vi "Create.vi"(6 "commandTimeout":i32, 8 "error in (no error)":errorcluster, 9 "DynamicParameters":refnum<class "DynamicParameters.lvclass">, 10 "tableName":string, 11 "SqlMapper in":refnum<class "SqlMapper.lvclass">) -> (0 "error out":errorcluster, 2 "id":variant, 3 "SqlMapper out":refnum<class "SqlMapper.lvclass">)   [LabVIEW 2020, in "ORM.lvlib" / "SqlMapper.lvclass"]
uses:
  SqlMapper.lvclass
  SqlMapper.lvclass/SqlMapper.ctl
  DbConnection/DbConnection.lvclass
  DynamicParameters/DynamicParameters.lvclass
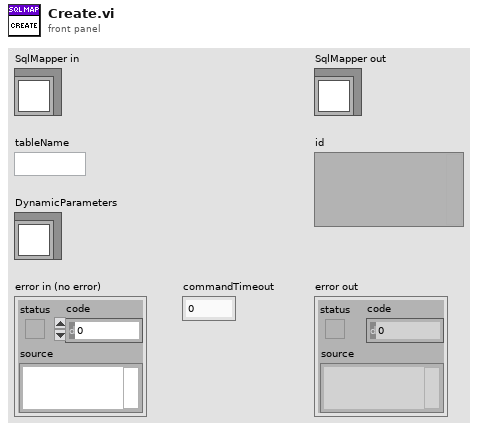
[diagram p1: front panel]
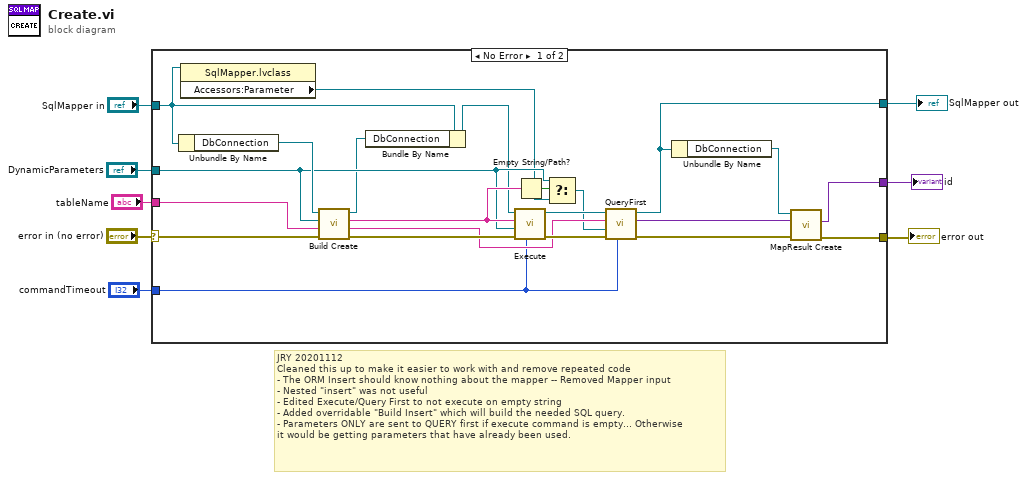
[diagram p0: block diagram]
diagram:
  # "JRY 20201112\nCleaned this up to make it easier to work with and remove repeated code\n- The ORM Insert should know nothing about the mapper -- Removed Mapper input\n- Nested \"insert\" was not useful\n- Edited Execute/Query First to not execute on empty string\n- Added overridable \"Build Insert\" which will build the needed SQL query.\n- Parameters ONLY are sent to QUERY first if execute command is empty... Otherwise\nit would be getting parameters that have already been used."
  n1 = case shown="No Error" "error in (no error)" {
    selector: "error in (no error)" -> [w30 w31]
    tunnel: "SqlMapper in" -> [w10 w32]
    tunnel: [w12 w32] -> w6
    tunnel: "DynamicParameters" -> [w16 _]
    tunnel: [w23 _] -> w4
    tunnel: [w21 w31] -> w3
    tunnel: "commandTimeout" -> [w15 _]
    tunnel: "tableName" -> [w20 _]
    frame No Error {
      n2 = Unbundle By Name(w10) -> ("DbConnection"=w25:refnum<class "DbConnection.lvclass">)
      n3 = property class="SqlMapper.lvclass"(reference=w10) -> ("Accessors:Parameter"=w9:refnum<class "DynamicParameters.lvclass">)  [unwired: 1 in, 2 out]
      n4 = call-dynamic "Build Create.vi"("error in (no error)"=w30, "tableName"=w20, "DynamicParameters in"=w16, "DbConnection in"=w25) -> ("error out"=w29:errorcluster, "LastIdentityQuery"=w26:string, "InsertStatement"=w19:string, "DbConnection out"=w13:refnum<class "DbConnection.lvclass">)  [unwired: 4 in]
      n5 = Bundle By Name(cluster=w10, "DbConnection"=w13) -> (w14:refnum<class "SqlMapper.lvclass">)
      n6 = call-dynamic "Execute.vi"("commandTimeout"=w15, "error in (no error)"=w29, "DynamicParameters"=w16, "sql"=w19, "SqlMapper in"=w14) -> ("error out"=w28:errorcluster, "SqlMapper out"=w27:refnum<class "SqlMapper.lvclass">)  [unwired: 4 in, 1 out]
      n7 = Empty String/Path?(string/path=w19) -> (empty?=w18:bool)
      n8 = Select(t=w16, s=w18, f=w9) -> (s? t:f=w17:refnum<class "DynamicParameters.lvclass">)
      n9 = call-dynamic "QueryFirst.vi"("commandTimeout in"=w15, "error in (no error)"=w28, "DynamicParameters in"=w17, "sql"=w26, "SqlMapper in"=w27) -> ("error out"=w22:errorcluster, "Value"=w24:variant, "SqlMapper out"=w12:refnum<class "SqlMapper.lvclass">)  [unwired: 4 in]
      n10 = Unbundle By Name(w12) -> ("DbConnection"=w11:refnum<class "DbConnection.lvclass">)
      n11 = call-dynamic "MapResult Create.vi"("error in (no error)"=w22, "InsertResultVariant"=w24, "DbConnection in"=w11) -> ("error out"=w21:errorcluster, "ID"=w23:variant)  [unwired: 7 in]
    }
    frame Error {
    }
  }
  "error out" <- w3
  "SqlMapper out" <- w6
  "id" <- w4
